vi "CFTS-Write Defaults.vi"(0 "AppName":string="CFTS\\CAPTH", 5 "Type of anything":variant, 7 "User":string, 11 "error in (no error)":errorcluster) -> (4 "Path out":path, 15 "error out":errorcluster)   [LabVIEW 2020]
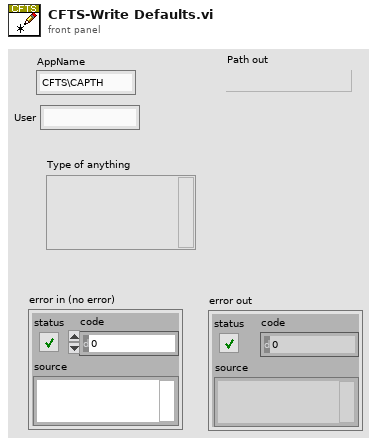
[diagram p1: front panel]
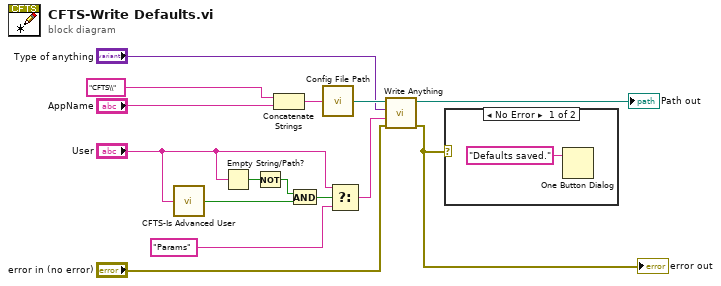
[diagram p0: block diagram]
diagram:
  n1 = call "CFTS-Is Advanced User.vi"("Experimenter"="User") -> ("Advanced user"=w7:bool)
  n2 = Empty String/Path?(string/path="User") -> (empty?=w4:bool)
  n3 = Not(x=w4) -> (.not. x?=w3:bool)
  n4 = Concatenate Strings("CFTS\\" ("string"), "AppName") -> (w12:string)
  n5 = And(x=w3, y=w7) -> (x .and. y?=w5:bool)
  n6 = call "Config File Path.vi"("AppName"=w12) -> ("Default config file name"=w15:path)
  n7 = Select(t="User", s=w5, f="Params") -> (s? t:f=w1:string)
  n8 = call "Write Anything.vi"("Error In"="error in (no error)", "Section Name (Name of \"Anything\")"=w1, "Anything"="Type of anything", "Path (dialog)"=w15) -> ("Error Out"=w8:errorcluster, "Path out"=→"Path out":path)  [unwired: 6 in]
  "error out" <- w8
  n9 = case shown="No Error" w8 {
    frame No Error {
      n10 = One Button Dialog(message="Defaults saved.") -> ()  [unwired: 1 in, 1 out]
    }
    frame Error {
    }
  }
